vi "RemoteControl.TestLauncher.ConnectionMonitor.vi"(8 "error in (no error)":errorcluster, 11 "RC Type":T2) -> (0 "error out":errorcluster)   [LabVIEW 2019, in "RemoteControl.lvclass"]
uses:
  RemoteControl.lvclass
  <vilib>/JKI/JKI SMO/SMO/SMO.lvclass
  <vilib>/JKI/JKI SMO/SMO/Typedefs/SMOState --Enum.ctl
  Typedefs/Message--Cluster.ctl
  Typedefs/PrivateEvents--RemoteControl.SendMessageToProcess.ctl
  C:/Program Files (x86)/National Instruments/LabVIEW 2019/vi.lib/JKI/JKI SMO/SMO/SMO.lvclass
  Typedefs/PrivateEvents--RemoteControl.Configure.ctl
  Typedefs/RC Com Type--enum.ctl
panel:
  in  "Debug Mode":bool
  in  "Check Timing Mode":bool
  out "processed":i32=809
  out "Message":T1
  in  "Configure":T3={"address"="*", "Port"=6341, "AllowedRemote"="", "Commands"=["Command1", "Command2", "Command3", "ACK", "HELP"]}
  out "SMO State":T4=enum."Stopped"
  in  "Stop":bool=TRUE
  # "SM SMO Test Launcher: Connection Monitor"
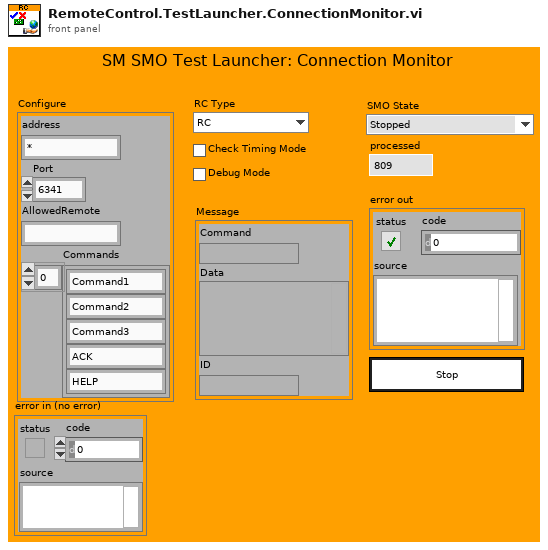
[diagram p1: front panel]
types:
  T1 = typedef "RemoteControl.lvclass/Message--Cluster.ctl" = cluster{"Command":string, "Data":variant, "ID":string}
  T2 = typedef "RemoteControl.lvclass/RC Com Type--enum.ctl" = enum16{"RC", "STM", "ZMQ"}
  T3 = typedef "RemoteControl.lvclass/PrivateEvents--RemoteControl.Configure.ctl" = cluster{"address":string, "Port":u16, "AllowedRemote":string, "Commands":string[]}
  T4 = typedef "SMO.lvclass/SMOState --Enum.ctl" = enum16{"unknown", "Created", "Started", "Stopped"}
  T5 = typedef "SMO.lvclass/Public Events.ctl" = cluster{"Error":refnum<user-event>, "State":refnum<user-event>, "Reserve State":refnum<user-event>}
  T6 = typedef "RemoteControl.lvclass/PublicEvents--Cluster.ctl" = cluster{"SendMessageFromProcess":refnum<user-event>}
  T7 = typedef "RemoteControl.lvclass/PrivateEvents--RemoteControl.SendMessageToProcess.ctl" = cluster{"Message":T1}
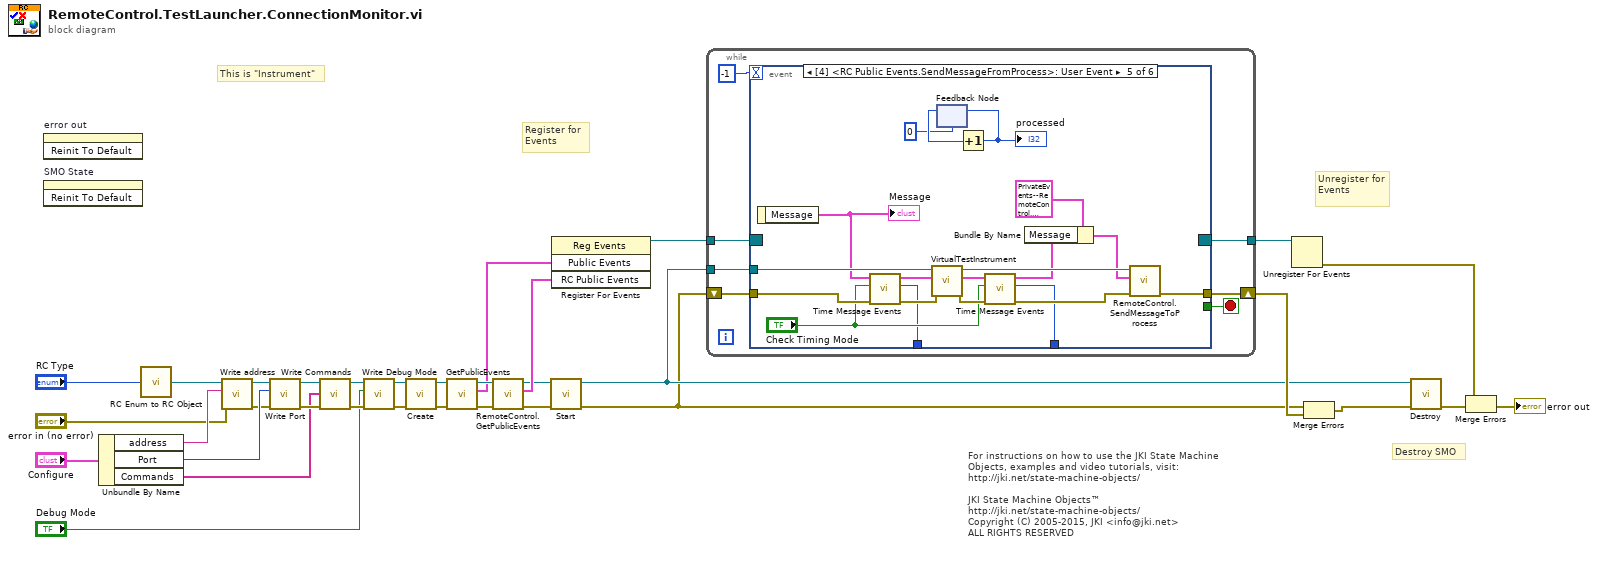
[diagram p0: block diagram]
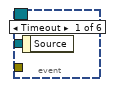
[diagram p2: hidden frame]
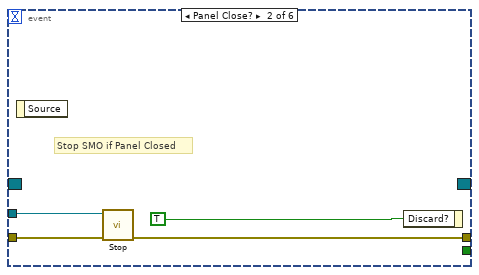
[diagram p3: hidden frame]
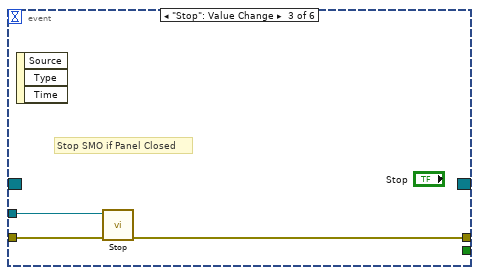
[diagram p4: hidden frame]
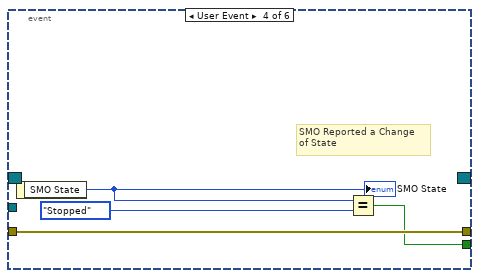
[diagram p5: hidden frame]
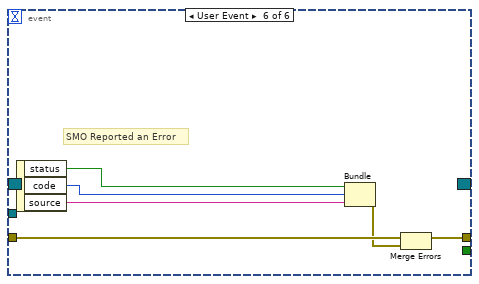
[diagram p6: hidden frame]
diagram:
  # "Register for Events"
  # "This is \"Instrument\""
  # "For instructions on how to use the JKI State Machine Objects, examples and video tutorials, visit:\nhttp://jki.net/state-machine-objects/\n\nJKI State Machine Objects™\nhttp://jki.net/state-machine-objects/\nCopyright (C) 2005-2015, JKI <info@jki.net>\nALL RIGHTS RESERVED"
  # "Destroy SMO"
  # "Unregister for Events"
  n1 = invoke on="error out" class="Clust (strict)" method="Reinit To Default"() -> ()  [unwired: 3 in, 3 out]
  n2 = invoke on="SMO State" class="Enum (strict)" method="Reinit To Default"() -> ()  [unwired: 3 in, 3 out]
  n3 = Unbundle By Name("Configure") -> ("address"=w15:string, "Port"=w14:u16, "Commands"=w9:string[])
  n4 = call "RC Enum to RC Object.vi"("RC Type"="RC Type") -> ("RemoteControl out"=w2:refnum<class "RemoteControl.lvclass">)
  n5 = call-dynamic "Write address.vi"("error in (no error)"="error in (no error)", "address"=w15, "RemoteControl in"=w2) -> ("error out"=w12:errorcluster, "RemoteControl out"=w13:refnum<class "RemoteControl.lvclass">)  [unwired: 7 in]
  n6 = call-dynamic "Write Port.vi"("error in (no error)"=w12, "Port"=w14, "RemoteControl in"=w13) -> ("error out"=w10:errorcluster, "RemoteControl out"=w11:refnum<class "RemoteControl.lvclass">)  [unwired: 7 in]
  n7 = call-dynamic "Write Commands.vi"("error in (no error)"=w10, "Commands"=w9, "RemoteControl in"=w11) -> ("error out"=w8:errorcluster, "RemoteControl out"=w7:refnum<class "RemoteControl.lvclass">)  [unwired: 7 in]
  n8 = call "Write Debug Mode.vi"("error in (no error)"=w8, "Debug Mode?"="Debug Mode", "RemoteControl in"=w7) -> ("error out"=w5:errorcluster, "RemoteControl out"=w6:refnum<class "RemoteControl.lvclass">)  [unwired: 7 in]
  n9 = call <vilib>:"Create.vi"("error in (no error)"=w5, "SMO"=w6) -> ("error out"=w28:errorcluster, "SMO out"=w20:refnum<class "RemoteControl.lvclass">)  [unwired: 7 in, 1 out]
  n10 = call <vilib>:"GetPublicEvents.vi"("error in (no error)"=w28, "SMO"=w20) -> ("error out"=w26:errorcluster, "Public Events"=w25:T5, "SMO out"=w27:refnum<class "RemoteControl.lvclass">)  [unwired: 7 in]
  n11 = call "RemoteControl.GetPublicEvents.vi"("error in (no error)"=w26, "RemoteControl"=w27) -> ("error out"=w22:errorcluster, "RC Public Events"=w23:T6, "RemoteControl out"=w21:refnum<class "RemoteControl.lvclass">)  [unwired: 7 in]
  n12 = call <vilib>:"Start.vi"("error in (no error)"=w22, "SMO"=w21) -> ("error out"=w18:errorcluster, "SMO out"=w19:refnum<class "RemoteControl.lvclass">)  [unwired: 8 in]
  n13 = register-events(w25, w23) -> (reference out=w24:refnum<event-registration>)  [unwired: 2 in, 1 out]
  n14 = while {
    shift-right: [w39] -> w32
    shift-left: w18 -> [w38]
    tunnel: w24 -> [w37]
    tunnel: [w36] -> w33
    tunnel: w19 -> [w35]
    stop <- w40 stop-if-true
    n15 = event shown="[4] <RC Public Events.SendMessageFromProcess>: User Event" {
      selector: w37 -> [_ _ _ _ _ _]
      dyn-events: [_ _ _ _ _ _] -> w36
      timeout: -1 -> [_ _ _ _ _ _]
      tunnel: [_ _ _ w48 _ _] -> w40
      tunnel: w35 -> [_ w44 w47 _ w65 _]
      tunnel: [_ w43 w46 w51 _ w74] -> w39
      tunnel: w38 -> [_ w42 w45 w51 w62 w72]
      tunnel: [_ _ _ _ w70 _] -> _
      tunnel: [_ _ _ _ w55 _] -> _
      tunnel: [_ _ _ _ w54 _] -> _
      event Timeout {
        n16 = event-data() -> ()  [unwired: 1 in, 1 out]
      }
      event Panel Close? {
        # "Stop SMO if Panel Closed"
        n17 = event-data() -> ()  [unwired: 1 in, 1 out]
        n18 = call <vilib>:"Stop.vi"("error in (no error)"=w42, "SMO"=w44) -> ("error out"=w43:errorcluster)  [unwired: 8 in, 1 out]
        n19 = event-data("Discard?"=TRUE ("OK")) -> ()  [unwired: 1 in, 1 out]
      }
      event "Stop": Value Change {
        # "Stop SMO if Panel Closed"
        n20 = event-data() -> ()  [unwired: 1 in, 3 out]
        n21 = call <vilib>:"Stop.vi"("error in (no error)"=w45, "SMO"=w47) -> ("error out"=w46:errorcluster)  [unwired: 8 in, 1 out]
      }
      event User Event {
        # "SMO Reported a Change\nof State"
        n22 = event-data() -> ("SMO State"=w50:T4)  [unwired: 1 in]
        "SMO State" <- w50
        n23 = Equal?(x=w50, y=SMOState_--Enum."Stopped") -> (x = y?=w48:bool)
      }
      event User Event {
        n24 = event-data() -> ("Message"=w63:T1)  [unwired: 1 in]
        "Message" <- w63
        n25 = call "Time Message Events.vi"("error in (no error)"=w62, "Debug Mode"="Check Timing Mode", "Message in"=w63) -> ("error out"=w61:errorcluster, "time (ms)"=w55:u32, "Message out"=w53:T1)  [unwired: 6 in]
        n26 = call "VirtualTestInstrument.vi"("error in (no error)"=w61, "Message"=w53, "RemoteControl"=w65) -> ("error out"=w58:errorcluster, "processed Message"=w52:T1, "RemoteControl"=w64:refnum<class "RemoteControl.lvclass">)  [unwired: 6 in]
        n27 = feedback #1(0) -> (w67:i32)
        n28 = Increment(x=w67) -> (x+1=w68:i32)
        "processed" <- w68
        n29 = feedback-in #1(w68) -> ()
        n30 = call "Time Message Events.vi"("error in (no error)"=w58, "Debug Mode"="Check Timing Mode", "Message in"=w52) -> ("error out"=w60:errorcluster, "time (ms)"=w54:u32, "Message out"=w57:T1)  [unwired: 6 in]
        n31 = Bundle By Name(cluster=T7 {"Message"={"Command"="", "Data"=variant(bool FALSE), "ID"=""}} ("SendMessgaeToProcess"), "Message"=w57) -> (w59:T7)
        n32 = call "RemoteControl.SendMessageToProcess.vi"("error in (no error)"=w60, "SendMessageToProcess"=w59, "RemoteControl"=w64) -> ("error out"=w70:errorcluster)  [unwired: 7 in, 1 out]
      }
      event User Event {
        # "SMO Reported an Error"
        n33 = event-data() -> ("status"=w73:bool, "code"=w76:i32, "source"=w75:string)  [unwired: 1 in]
        n34 = Bundle("status"=w73, "code"=w76, "source"=w75) -> (w71:errorcluster)  [unwired: 1 in]
        n35 = Merge Errors(w72, w71) -> (w74:errorcluster)
      }
    }
  }
  n36 = Unregister For Events(event registration refnum=w33) -> (error out=w31:errorcluster)  [unwired: 1 in]
  n37 = Merge Errors(w18, w32) -> (w17:errorcluster)
  n38 = call <vilib>:"Destroy.vi"("error in (no error)"=w17, "SMO"=w19) -> ("error out"=w29:errorcluster)  [unwired: 9 in]
  n39 = Merge Errors(w31, w29) -> (→"error out":errorcluster)
